vi "Configure Measurements.vi"(0 "VISA resource name":refnum<visa-resource-name>, 5 "Measurement (0: Voltage Channel 1)":i32(ring) items=["Voltage Channel 1", "Voltage Channel 2", "Temperature Channel 1", "Temperature Channel 2"], 7 "Integration Rate (5)":dbl=5.0, 9 "Integration Rate Units (0: Line Cycles)":i32(ring) items=["Line Cycles", "Seconds"], 11 "error in (no error)":errorcluster, 12 "Sample Count (1)":i32=1) -> (4 "VISA resource name out":refnum<visa-resource-name>, 15 "error out":errorcluster)   [LabVIEW 2011, in "Keithley 2182.lvlib"]
doc: "Configures the type of measurement to perform."
uses:
  Keithley 2182.lvlib
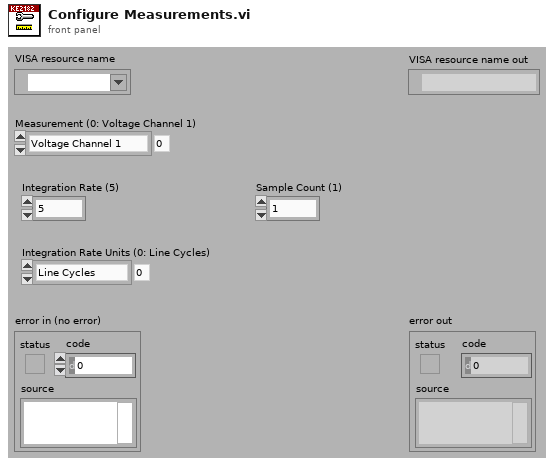
[diagram p1: front panel]
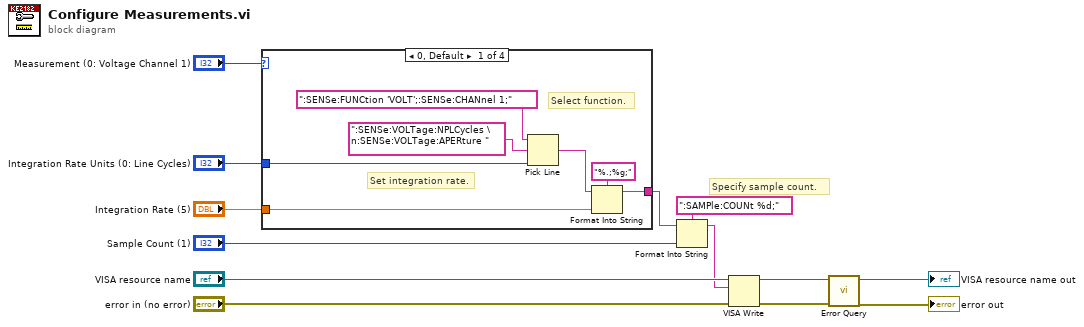
[diagram p0: block diagram]
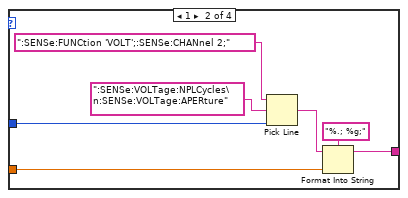
[diagram p2: hidden frame]
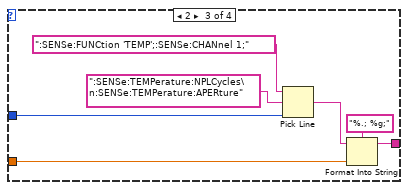
[diagram p3: hidden frame]
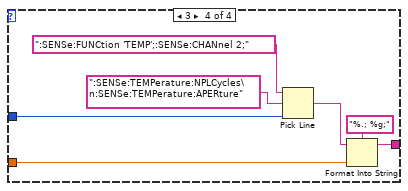
[diagram p4: hidden frame]
diagram:
  # "Specify sample count."
  n1 = case shown="0, Default" "Measurement (0: Voltage Channel 1)" {
    tunnel: [w14 w21 w29 w36] -> w3
    tunnel: "Integration Rate Units (0: Line Cycles)" -> [w17 w24 w32 w39]
    tunnel: "Integration Rate (5)" -> [w15 w22 w30 w37]
    frame 0, Default {
      # "Select function."
      # "Set integration rate."
      n2 = Pick Line(string ("")=":SENSe:FUNCtion 'VOLT';:SENSe:CHANnel 1;", multi-line string=":SENSe:VOLTage:NPLCycles \n:SENSe:VOLTage:APERture ", line index=w17) -> (output string=w16:string)
      n3 = Format Into String(format string="%.;%g;", initial string=w16, w15) -> (resulting string=w14:string)  [unwired: 1 in, 1 out]
    }
    frame 1 {
      n4 = Pick Line(string ("")=":SENSe:FUNCtion 'VOLT';:SENSe:CHANnel 2;", multi-line string=":SENSe:VOLTage:NPLCycles\n:SENSe:VOLTage:APERture", line index=w24) -> (output string=w23:string)
      n5 = Format Into String(format string="%.; %g;", initial string=w23, w22) -> (resulting string=w21:string)  [unwired: 1 in, 1 out]
    }
    frame 2 {
      n6 = Pick Line(string ("")=":SENSe:FUNCtion 'TEMP';:SENSe:CHANnel 1;", multi-line string=":SENSe:TEMPerature:NPLCycles\n:SENSe:TEMPerature:APERture", line index=w32) -> (output string=w31:string)
      n7 = Format Into String(format string="%.; %g;", initial string=w31, w30) -> (resulting string=w29:string)  [unwired: 1 in, 1 out]
    }
    frame 3 {
      n8 = Pick Line(string ("")=":SENSe:FUNCtion 'TEMP';:SENSe:CHANnel 2;", multi-line string=":SENSe:TEMPerature:NPLCycles\n:SENSe:TEMPerature:APERture", line index=w39) -> (output string=w38:string)
      n9 = Format Into String(format string="%.; %g;", initial string=w38, w37) -> (resulting string=w36:string)  [unwired: 1 in, 1 out]
    }
  }
  n10 = Format Into String(format string=":SAMPle:COUNt %d;", initial string=w3, "Sample Count (1)") -> (resulting string=w1:string)  [unwired: 1 in, 1 out]
  n11 = VISA Write(VISA resource name="VISA resource name", write buffer=w1, error in (no error)="error in (no error)") -> (VISA resource name out=w11:refnum<visa-resource-name>, error out=w10:errorcluster)  [unwired: 1 out]
  n12 = call "Error Query.vi"("error in (no error)"=w10, "VISA resource name"=w11) -> ("error out"=→"error out":errorcluster, "VISA resource name out"=→"VISA resource name out":refnum<visa-resource-name>)  [unwired: 6 in, 2 out]
